vi "WM New Hampshire Typical.vi"(0 "Significant Wave Height":dbl=1.21 min=0.0 step=0.01 format="%.2f", 1 "Gamma 1":dbl=6.75 format="%.2f", 2 "Gamma 2":dbl=0.5 format="%.2f", 3 "Start Freq (Model Scale)":dbl format="%.2f", 5 "Peak Wave Period 1":dbl=10.0 min=0.0 step=0.01 format="%.2f", 7 "Peak Wave Period 2":dbl=5.34 min=-1.0 max=9.0 format="%.2f", 9 "Scale Ratio":dbl=15.2 format="%.2f", 11 "P":dbl=4.35 format="%.2f", 12 "Number of Frequencies":i32=2 min=2, 14 "End Freq (Model Scale)":dbl=100.0 format="%.2f") -> (6 "NH Typical parameters":T1 {"Sig Wave Period 2" format="%.2f"; "Scale Ratio" format="%.2f"; "P" format="%.2f"; "Gamma 2" format="%.2f"; "Gamma 1" format="%.2f"; "Sig Wave Period" format="%.2f"; "Sig Wave Height" format="%.2f"}, 10 "Spectral Energy":dbl[](array[numeric]) format="%.2f", 15 "Frequency":dbl[](array[numeric]) caption="Hz" format="%.2f")   [LabVIEW 2012]
panel:
  in  "Boolean":bool
  # "New Hampshire Typical Wave Spectra"
  # "m  (Full Scale)"
  # "s  (Full Scale)"
  # "s  (Full Scale)"
  # ":1"
  # "Full Scale : Model Scale"
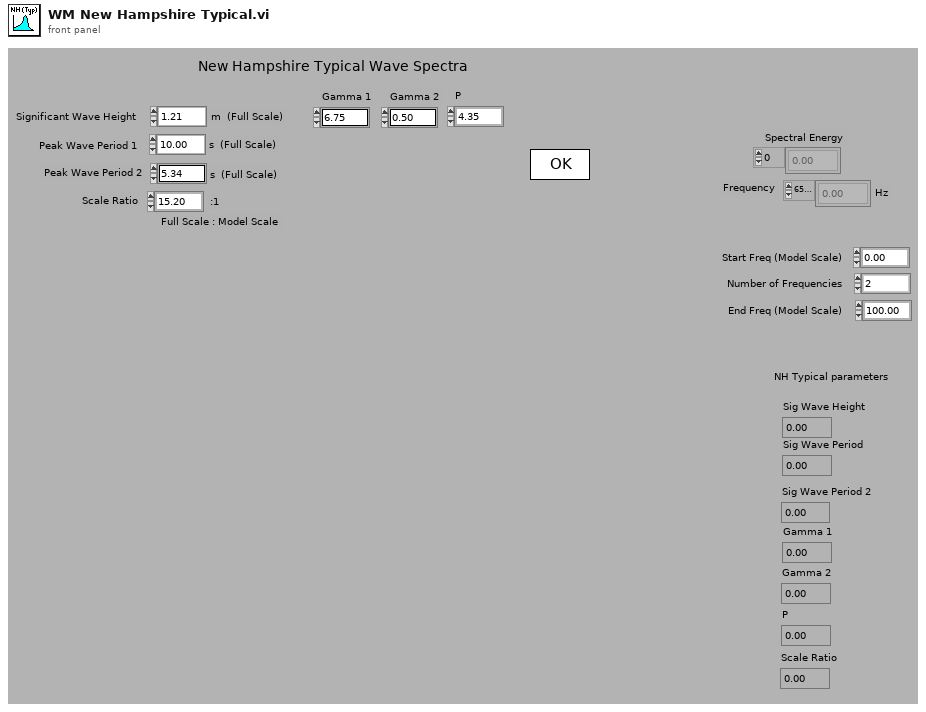
[diagram p1: front panel]
types:
  T1 = cluster{"Sig Wave Height":dbl, "Sig Wave Period":dbl, "Sig Wave Period 2":dbl, "Gamma 1":dbl, "Gamma 2":dbl, "P":dbl, "Scale Ratio":dbl}
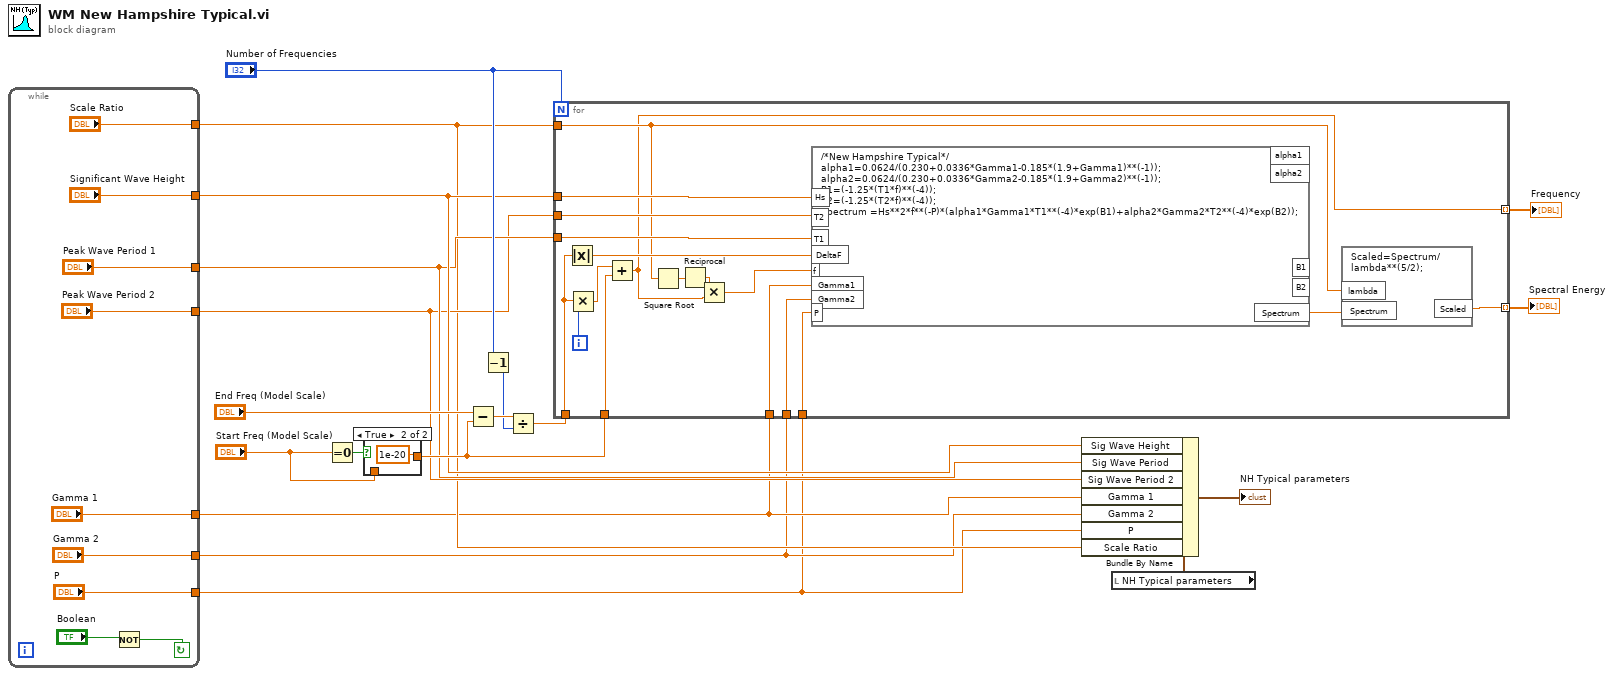
[diagram p0: block diagram]
diagram:
  n1 = while {
    tunnel: ["P"] -> w2
    tunnel: ["Gamma 2"] -> w3
    tunnel: ["Gamma 1"] -> w4
    tunnel: ["Scale Ratio"] -> w5
    tunnel: ["Peak Wave Period 2"] -> w6
    tunnel: ["Peak Wave Period 1"] -> w7
    tunnel: ["Significant Wave Height"] -> w8
    stop <- w20 continue-if-true
    n2 = Not(x="Boolean") -> (.not. x?=w20:bool)
  }
  n3 = Equal To 0?(x="Start Freq (Model Scale)") -> (x = 0?=w13:bool)
  n4 = case shown="True" w13 {
    tunnel: [w29 1e-20] -> w11
    tunnel: "Start Freq (Model Scale)" -> [w29 _]
    frame False {
    }
    frame True {
    }
  }
  n5 = Subtract(x="End Freq (Model Scale)", y=w11) -> (x-y=w17:dbl)
  n6 = Decrement(x="Number of Frequencies") -> (x-1=w15:i32)
  n7 = Divide(x=w17, y=w15) -> (x/y=w16:dbl)
  n8 = for {
    N: "Number of Frequencies" -> [_]
    tunnel: w8 -> [w44]
    tunnel: w7 -> [w45]
    tunnel: [w31] -> w1 mode=indexing
    tunnel: [w36] -> w19 mode=indexing
    tunnel: w11 -> [w42]
    tunnel: w16 -> [w47]
    tunnel: w4 -> [w40]
    tunnel: w3 -> [w39]
    tunnel: w6 -> [w41]
    tunnel: w2 -> [w38]
    tunnel: w5 -> [w35]
    i -> [w48]
    n9 = Absolute Value(x=w47) -> (abs(x)=w46:dbl)
    n10 = Multiply(x=w47, y=w48) -> (x*y=w43:dbl)
    n11 = Add(x=w43, y=w42) -> (x+y=w31:dbl)
    n12 = Square Root(x=w35) -> (sqrt(x)=w34:dbl)
    n13 = Reciprocal(x=w34) -> (1/x=w33:dbl)
    n14 = Multiply(x=w33, y=w31) -> (x*y=w32:dbl)
    n15 = formula code="/*New Hampshire Typical*/\nalpha1=0.0624/(0.230+0.0336*Gamma1-0.185*(1.9+Gamma1)**(-1));\nalpha2=0.0624/(0.230+0.0336*Gamma2-0.185*(1.9+Gamma2)**(-1));\nB1=(-1.25*(T1*f)**(-4));\nB2=(-1.25*(T2*f)**(-4));\nSpectrum =Hs**2*f**(-P)*(alpha1*Gamma1*T1**(-4)*exp(B1)+alpha2*Gamma2*T2**(-4)*exp(B2));"("Hs"=w44, "T1"=w45, "f"=w32, "DeltaF"=w46, "Gamma1"=w40, "Gamma2"=w39, "T2"=w41, "P"=w38) -> ("Spectrum"=w37:dbl)  [unwired: 4 out]
    n16 = formula code="Scaled=Spectrum/lambda**(5/2);"("lambda"=w35, "Spectrum"=w37) -> ("Scaled"=w36:dbl)
  }
  "Spectral Energy" <- w19
  "Frequency" <- w1
  n17 = local read "NH Typical parameters"() -> (w10:T1)
  n18 = Bundle By Name(cluster=w10, "Sig Wave Height"=w8, "Sig Wave Period"=w7, "Sig Wave Period 2"=w6, "Gamma 1"=w4, "Gamma 2"=w3, "P"=w2, "Scale Ratio"=w5) -> (→"NH Typical parameters":T1)
